vi "SaveVernierCalibV1729A.vi"(8 "error in (no error)":errorcluster, 9 "Group Name":string="Calibration", 10 "VernierCals":T1, 11 "File Handle":T2 format="%.0x") -> (0 "error out":errorcluster)   [LabVIEW 2014]
uses:
  <vilib>/addons/h5labview2/base/hid_t.ctl
  <vilib>/addons/h5labview2/base/lib_path.vi
  <vilib>/addons/h5labview2/base/H5Equery.vi
  <vilib>/addons/h5labview2/dataset/H5Dwrite.llb/H5Dwrite.xnode
  <vilib>/addons/h5labview2/group/H5G.lvlib
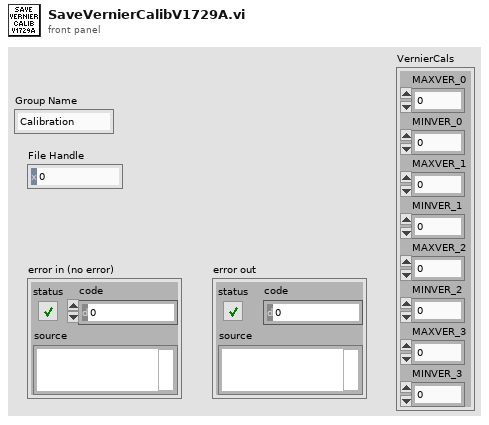
[diagram p1: front panel]
types:
  T1 = cluster{"MAXVER_0":u16, "MINVER_0":u16, "MAXVER_1":u16, "MINVER_1":u16, "MAXVER_2":u16, "MINVER_2":u16, "MAXVER_3":u16, "MINVER_3":u16}
  T2 = typedef "hid_t.ctl" = i32
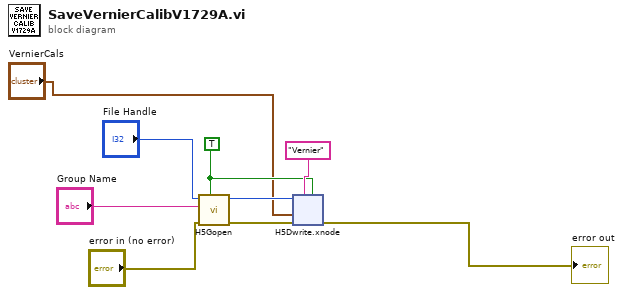
[diagram p0: block diagram]
diagram:
  w3 = TRUE ("create? (F)")
  n1 = call <vilib>:"H5Gopen.vi"("create? (F)"=w3, "error in (no error)"="error in (no error)", "name"="Group Name", "ref in"="File Handle") -> ("error out"=w6:errorcluster, "group out"=w4:T2)  [unwired: 6 in]
  n2 = xnode "H5Dwrite.xnode"("replace? (F)"=w3, "dataset name"="Vernier", "error in (no error)"=w6, "data"="VernierCals", "ref in"=w4) -> ("error out"=→"error out":errorcluster)  [unwired: 2 in, 2 out]
